vi "MT Generate CPM System Parameters (Map).vi"(0 "samples per symbol (16)":i32=16, 5 "symbol indices":i32[][](array[numeric]), 7 "modulation index, h(i)":cluster{"numerator":i32, "denominator":i32}[](array[cluster]), 9 "symbol rate":dbl=1.0, 11 "error in (no error)":errorcluster) -> (6 "CPM system parameters":T1, 15 "error out":errorcluster)   [LabVIEW 2020, in "niDMT.lvlib"]
doc: "Calculates parameters for use with either the MT Modulate CPM VI or the MT Demodulate CPM VI. Wire the <B>CPM system parameters</B> passed from this VI to the corresponding cluster of the MT Modulate CPM, MT Demodulate CPM, and MT Detect CPM VIs. It accepts an input array of symbol values that explicitly define the positions of the symbol map."
uses:
  <vilib>/addons/Modulation/niDMT.lvlib
  <vilib>/addons/Modulation/Digital/Support/Controls/CPM System Parameters.ctl
  <vilib>/Analysis/1siggen.llb/Ramp Pattern by Samples.vi
  <vilib>/addons/Modulation/niAMT.lvlib
  <vilib>/Analysis/NI_AALBase.lvlib
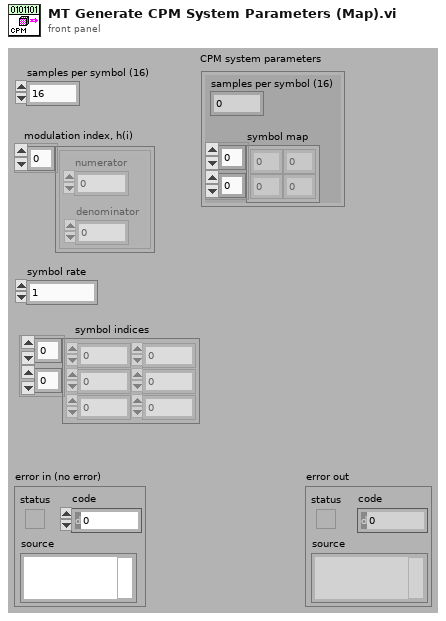
[diagram p1: front panel]
types:
  T1 = typedef "niDMT.lvlib/CPM System Parameters.ctl" = cluster{"samples per symbol (16)":i32, "symbol map":dbl[][]}
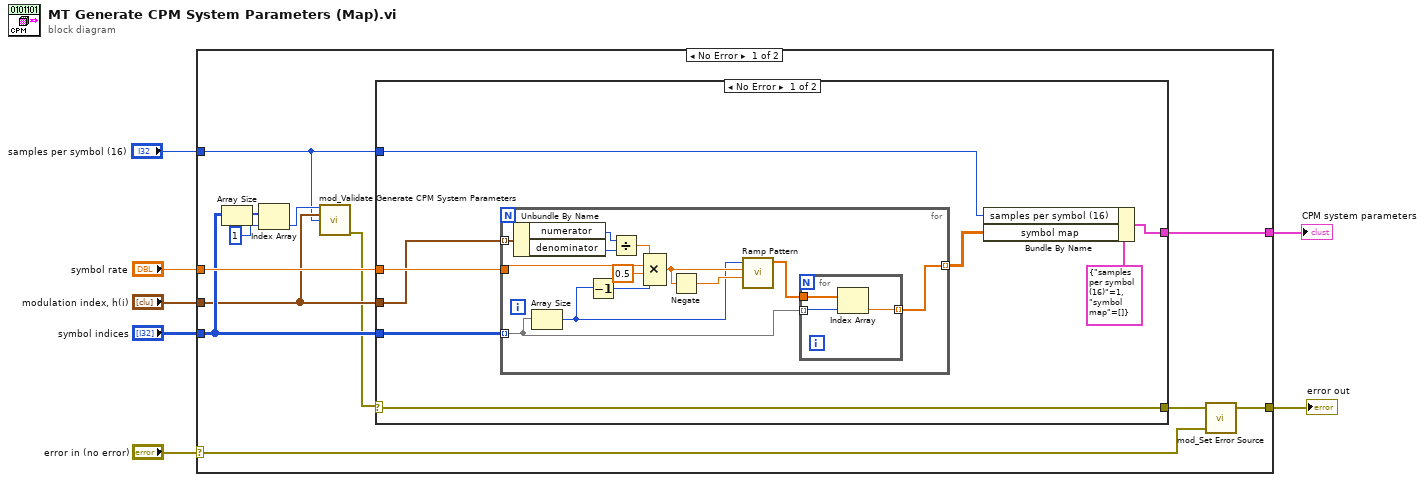
[diagram p0: block diagram]
diagram:
  n1 = case shown="No Error" "error in (no error)" {
    selector: "error in (no error)" -> [w9 w45]
    tunnel: "samples per symbol (16)" -> [w10 _]
    tunnel: [w16 _] -> w6
    tunnel: [w19 w45] -> w4
    tunnel: "modulation index, h(i)" -> [w11 _]
    tunnel: "symbol rate" -> [w17 _]
    tunnel: "symbol indices" -> [w15 _]
    frame No Error {
      n2 = Array Size(array=w15) -> (size(s)=w14:i32[])
      n3 = Index Array(array=w14, index=1) -> (element=w12:i32)
      n4 = call <vilib>:"mod_Validate Generate CPM System Parameters.vi"("M-CPM"=w12, "modulation index, h(i)"=w11, "samples per symbol"=w10) -> ("error out"=w8:errorcluster)  [unwired: 12 out]
      n5 = case shown="No Error" w8 {
        selector: w8 -> [w27 w44]
        tunnel: w10 -> [w20 _]
        tunnel: [w27 w44] -> w18
        tunnel: w11 -> [w24 _]
        tunnel: w17 -> [w25 _]
        tunnel: [w23 _] -> w16
        tunnel: w15 -> [w22 _]
        frame No Error {
          n6 = for {
            tunnel: w24 -> [w40] mode=indexing
            tunnel: w25 -> [w35]
            tunnel: [w30] -> w21 mode=indexing
            tunnel: w22 -> [w29] mode=indexing
            n7 = Unbundle By Name(w40) -> ("numerator"=w38:i32, "denominator"=w37:i32)
            n8 = Array Size(array=w29) -> (size(s)=w28:i32)
            n9 = Decrement(x=w28) -> (x-1=w32:i32)
            n10 = Divide(x=w38, y=w37) -> (x/y=w36:dbl)
            n11 = Compound Arithmetic op=MULTIPLY(w36, w35, 0.5 ("value"), w32) -> (w33:dbl)
            n12 = Negate(x=w33) -> (-x=w39:dbl)
            n13 = call-poly <vilib>:"Ramp Pattern.vi"("start"=w39, "end"=w33, "samples"=w28) -> ("Ramp Pattern"=w31:dbl[])  [unwired: 7 in, 1 out]
            n14 = for {
              tunnel: w31 -> [w43]
              tunnel: w29 -> [w42] mode=indexing
              tunnel: [w41] -> w30 mode=indexing
              n15 = Index Array(array=w43, index=w42) -> (element=w41:dbl)
            }
          }
          n16 = Bundle By Name(cluster=T1 {"samples per symbol (16)"=1, "symbol map"=[]} ("CPM system parameters"), "samples per symbol (16)"=w20, "symbol map"=w21) -> (w23:T1)
        }
        frame Error {
        }
      }
      n17 = call <vilib>:"mod_Set Error Source.vi"("initial error in (no error)"=w9, "final error in (no error)"=w18) -> ("error out"=w19:errorcluster)  [unwired: 3 out]
    }
    frame Error {
    }
  }
  "CPM system parameters" <- w6
  "error out" <- w4
